vi "Launch Elastic Module.vi"() -> ()   [LabVIEW 2016]
uses:
  Elastic Moduli.lvclass
  C:/github/LabActor/Template Module/Template Module.lvclass
  C:/Program Files (x86)/National Instruments/LabVIEW 2016/vi.lib/ActorFramework/Actor/Actor.lvclass
  Template Module/Template Module.lvclass/Template Module.ctl
  <vilib>/ActorFramework/Message Enqueuer/Message Enqueuer.lvclass/Message Enqueuer.ctl
  Template Module/Write Name.vi
  <vilib>/ActorFramework/Message Enqueuer/Enqueue.vi
  Template Module Messages/Open Front Panel Msg/Open Front Panel Msg.lvclass
  C:/Program Files (x86)/National Instruments/LabVIEW 2016/vi.lib/ActorFramework/Message/Message.lvclass
  <vilib>/ActorFramework/Message Priority Queue/Priority Enqueue.vi
  <vilib>/ActorFramework/Actor/Actor.lvclass
panel:
  out "Waiting Lights":T1
  out "Current action:":string
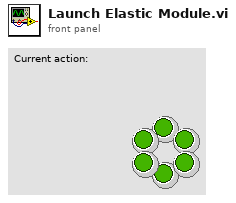
[diagram p1: front panel]
types:
  T1 = cluster{"DNL_wait 1":bool, "DNL_wait 1":bool, "DNL_wait 1":bool, "DNL_wait 1":bool, "DNL_wait 1":bool, "DNL_wait 1":bool}
  T2 = cluster{"[0]":bool, "[1]":bool, "[2]":bool, "[3]":bool, "[4]":bool, "[5]":bool}
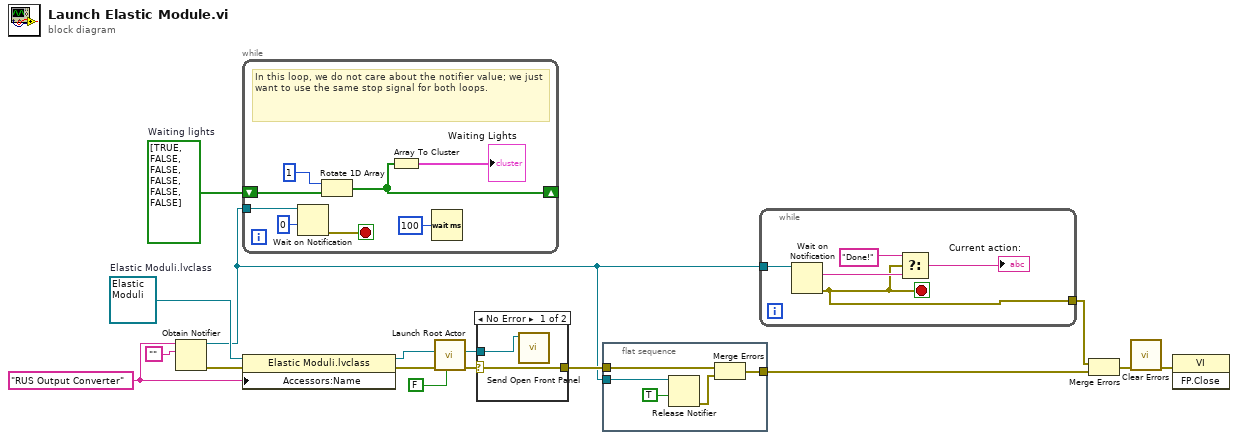
[diagram p0: block diagram]
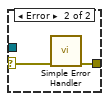
[diagram p2: hidden frame]
diagram:
  w11 = refnum<class "Elastic Moduli.lvclass"> refnum  # Elastic Moduli.lvclass
  w1 = "RUS Output Converter" ("Name")
  w12 = bool[] [TRUE, FALSE, FALSE, FALSE, FALSE, FALSE]  # Waiting lights
  n1 = Obtain Notifier(name (unnamed)=w1, notification data type="") -> (notifier out=w3:refnum<notifier>, error out=w10:errorcluster)  [unwired: 2 in, 1 out]
  n2 = while {
    shift-right: [w18] -> _
    shift-left: w12 -> [w20]
    tunnel: w3 -> [w22]
    stop <- w24 stop-if-true
    # "In this loop, we do not care about the notifier value; we just want to use the same stop signal for both loops."
    n3 = Wait on Notification(notifier=w22, timeout in ms (-1)=0) -> (error out=w24:errorcluster)  [unwired: 2 in, 3 out]
    n4 = Rotate 1D Array(1:w20, 2:1 ("n")) -> (0:w18:bool[])
    n5 = Array To Cluster(array=w18) -> (cluster=→"Waiting Lights":T2)
    n6 = Wait (ms)(milliseconds to wait=u32 100) -> ()  [unwired: 1 out]
  }
  n7 = property class="Elastic Moduli.lvclass"(reference=w11, error in=w10, "Accessors:Name"=w1) -> (reference out=w9:refnum<class "Elastic Moduli.lvclass">, error out=w8:errorcluster)
  n8 = call <vilib>:"Launch Root Actor.vi"("Open Actor Core front panel? (F)"=FALSE, "error in (no error)"=w8, "Actor"=w9) -> ("error out"=w6:errorcluster, "Actor's Enqueuer"=w5:refnum<class "Message Enqueuer.lvclass">)  [unwired: 7 in]
  n9 = case shown="No Error" w6 {
    selector: w6 -> [w26 w28]
    tunnel: [w26 w27] -> w4
    tunnel: w5 -> [w25 _]
    frame No Error {
      n10 = call "Send Open Front Panel.vi"("Message Enqueuer"=w25) -> ()  [unwired: 9 in, 2 out]
    }
    frame Error {
      n11 = call <vilib>:"Simple Error Handler.vi"("error in (no error)"=w28) -> ("error out"=w27:errorcluster)  [unwired: 4 in, 4 out]
    }
  }
  n12 = flat-sequence {
    tunnel: w4 -> [w31]
    tunnel: w3 -> [w32]
    tunnel: [w29] -> w2
    frame #0 {
      n13 = Release Notifier(notifier=w32, force destroy? (F)=TRUE ("Kill notifier")) -> (error out=w30:errorcluster)  [unwired: 1 in, 2 out]
      n14 = Merge Errors(w31, w30) -> (w29:errorcluster)
    }
  }
  n15 = while {
    tunnel: w3 -> [w38]
    tunnel: [w34] -> w13
    stop <- w34 stop-if-true
    n16 = Wait on Notification(notifier=w38) -> (notification=w36:string, error out=w34:errorcluster)  [unwired: 3 in, 2 out]
    n17 = Select(t="Done!" ("notification"), s=w34, f=w36) -> (s? t:f=→"Current action:":string)
  }
  n18 = Merge Errors(w13, w2) -> (w14:errorcluster)
  n19 = call <vilib>:"Clear Errors.vi"("error in (no error)"=w14) -> ("error out"=w16:errorcluster)  [unwired: 5 in, 1 out]
  n20 = invoke class="VI" method="FP.Close"(error in=w16) -> ()  [unwired: 2 in, 3 out]
